vi "FTW-Ether-Connections-Add.vi"(0 "Connection":string, 5 "Address":string, 11 "error in":errorcluster) -> (15 "error out":errorcluster)   [LabVIEW 2013, in "FTW-Ether.lvclass"]
uses:
  FTW-Ether.lvclass
  FTW-Ether-Connections-Action.ctl
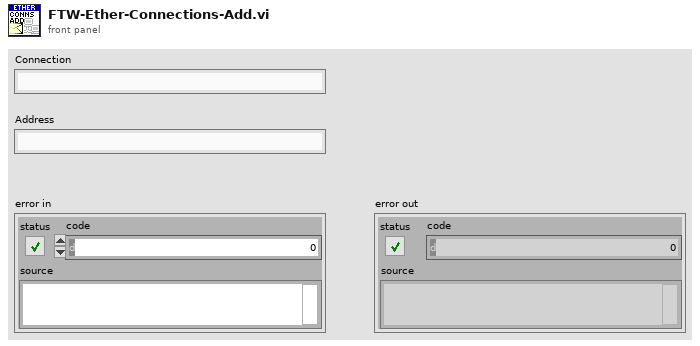
[diagram p1: front panel]
types:
  T1 = typedef "FTW-Ether.lvclass/FTW-Ether-Connections-Action.ctl" = enum8{"Query", "Add", "Reset"}
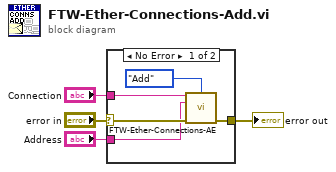
[diagram p0: block diagram]
diagram:
  n1 = case shown="No Error" "error in" {
    selector: "error in" -> [w9 w10]
    tunnel: [w8 w10] -> w3
    tunnel: "Connection" -> [w7 _]
    tunnel: "Address" -> [w6 _]
    frame No Error {
      n2 = call "FTW-Ether-Connections-AE.vi"("Connection"=w7, "Action"=FTW-Ether-Connections-Action."Add", "Address"=w6, "error in"=w9) -> ("error out"=w8:errorcluster)  [unwired: 10 in, 1 out]
    }
    frame Error {
    }
  }
  "error out" <- w3
